vi "Aircraft Yaw Stability.vi"() -> ()   [LabVIEW 2022 SP3]
doc: "This example demonstrates how to continuously acquire buffered voltage measurements using a DAQmx device.\n\nFor instructions on how to connect your signals to the DAQ device, refer to your device documentation."
uses:
  <vilib>/Utility/error.llb/DialogType.ctl
  <vilib>/DAQmx/read.llb/DAQmx Read (Analog 1D Wfm NChan NSamp).vi
  <vilib>/DAQmx/create/channels.llb/DAQmx Create Channel (AI-Voltage-Basic).vi
  <vilib>/DAQmx/configure/timing.llb/DAQmx Timing (Sample Clock).vi
  <vilib>/DAQmx/configure/task.llb/DAQmx Configure Logging (TDMS).vi
  <vilib>/DAQmx/configure/trigger.llb/DAQmx Start Trigger (Digital Edge).vi
  <vilib>/DAQmx/configure/trigger.llb/DAQmx Start Trigger (Time).vi
  <vilib>/DAQmx/configure/trigger.llb/DAQmx Start Trigger (Analog Edge).vi
  <vilib>/DAQmx/miscellaneous.llb/DAQmx Fill In Error Info.vi
  <resource>/objmgr/daqmx.rc
panel:
  in  "File Name":string="Group1"
  in  "Folder":path=path "S:/Research/EnFlo_Data_Current/2024/A_Tunnel/UG Labs/Results/Res_12-2024"
  in  "Trigger Type":T1(tab)
  in  "Digital Start Trigger Edge":i32(ring)=10280 caption="Edge" items=["Rising"=10280, "Falling"=10171]
  in  "Digital Start Trigger Source":tag="/Dev1/PFI0" caption="Source"
  in  "Digital Pause Trigger Pause When":i32(ring)=10192 caption="Pause When" items=["High"=10192, "Low"=10214]
  in  "Digital Pause Trigger Source":tag="/Dev1/PFI0" caption="Source"
  in  "Analog Start Trigger Level":dbl caption="Level" format="%0.2f"
  in  "Analog Start Trigger Hysteresis":dbl caption="Hysteresis" format="%.2f"
  in  "Analog Start Trigger Slope":i32(ring)=10280 caption="Slope" items=["Rising"=10280, "Falling"=10171]
  in  "Analog Start Trigger Source":string="APFI0" caption="Source"
  in  "Analog Pause Trigger Source":string="APFI0" caption="Source"
  in  "Analog Pause Trigger Pause When":i32(ring)=10093 caption="Pause When" items=["Above Level"=10093, "Below Level"=10107]
  in  "Analog Pause Trigger Level":dbl caption="Level" format="%.2f"
  in  "When":timestamp
  in  "Select Time\nManually":bool
  in  "Stop":bool
  out "Waveform Chart":waveform(dbl)[](graph)
  in  "TDMS File Path":path
  in  "Number of Samples":i32=100
  in  "Sample Rate":dbl=1000.0
  in  "Sample Clock Source":tag="OnboardClock"
  in  "Terminal Configuration":i32(ring)=-1 items=["default"=-1, "RSE"=10083, "NRSE"=10078, "Differential"=10106, "Pseudodifferential"=12529]
  in  "Max Voltage":dbl=10.0
  in  "Min Voltage":dbl=-10.0
  in  "Physical Channel":tag="Dev1/ai0"
  out "Actual Sample Rate":dbl=1000.0 format="%0.2f"
  in  "Logging Mode":i32(ring)=10231 items=["Off"=10231, "Log and Read"=15842]
  # "Channel Settings"
  # "Timing Settings"
  # "Trigger Settings"
  # "Logging Settings"
  # "To enable triggers, select a tab above, and configure the settings.\n\nNot all hardware supports all trigger types. Refer to your device documentation for more information."
  # "This trigger type is not supported in continuous sample timing. \n\nRefer to your device documentation for more information on which triggers are supported."
  # "This trigger type is not supported in continuous sample timing. \n\nRefer to your device documentation for more information on which triggers are supported."
  # "If time is not manually set, task will begin after 10 seconds"
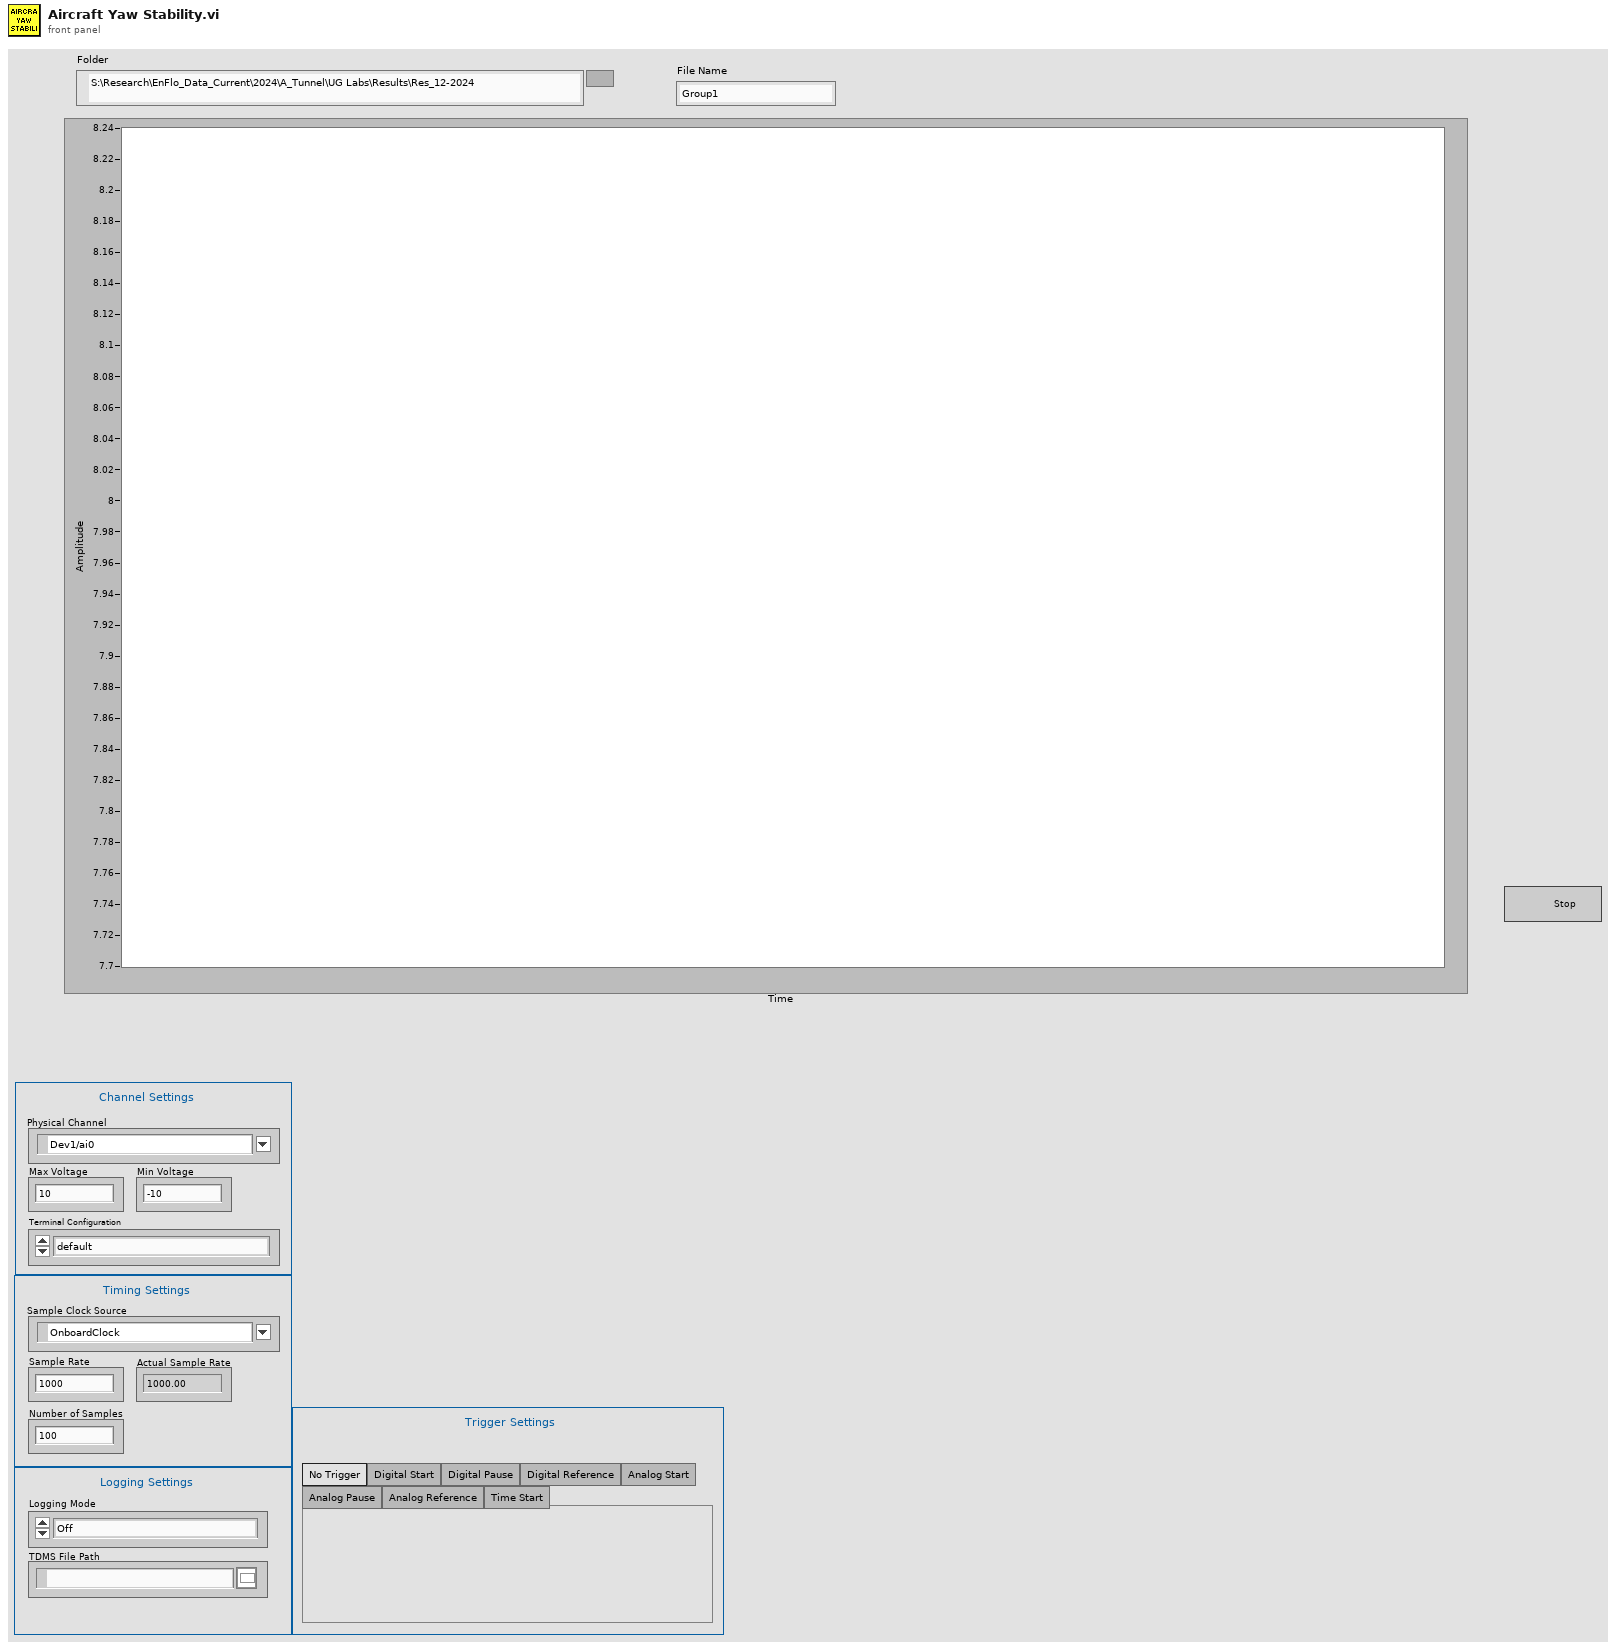
[diagram p1: front panel]
types:
  T1 = enum32{"No Trigger", "Digital Start", "Digital Pause", "Digital Reference", "Analog Start", "Analog Pause", "Analog Reference", "Time Start"}
  T2 = typedef "DialogType.ctl" = u16
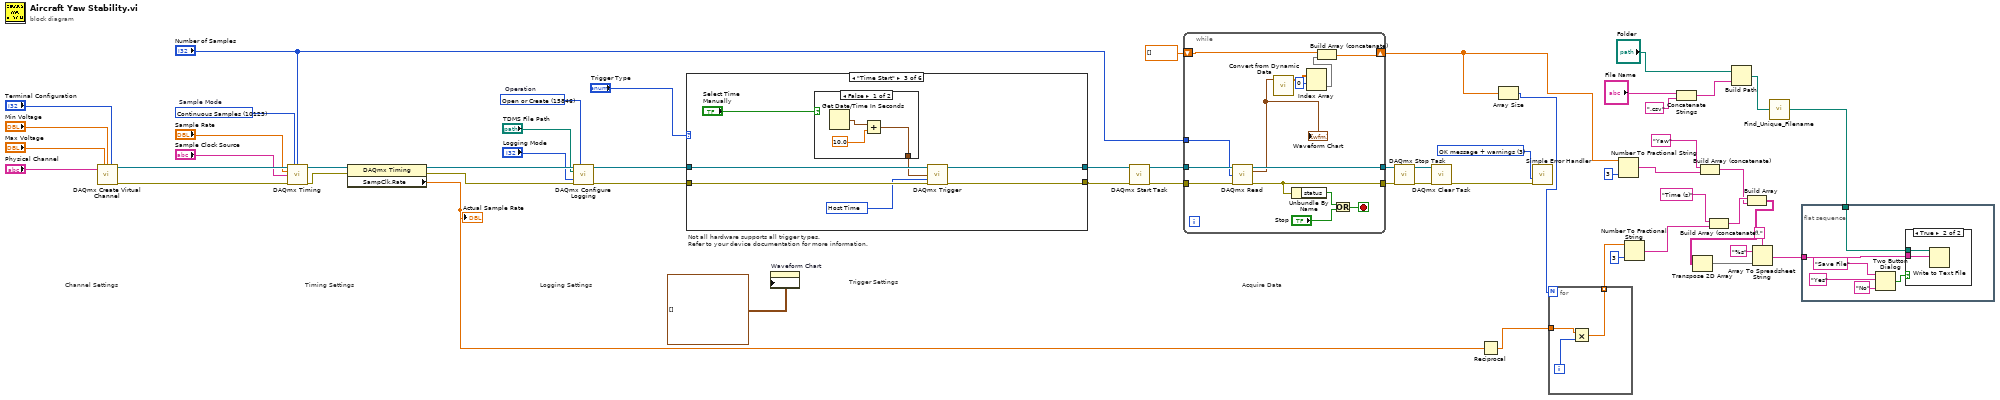
[diagram p0: block diagram]
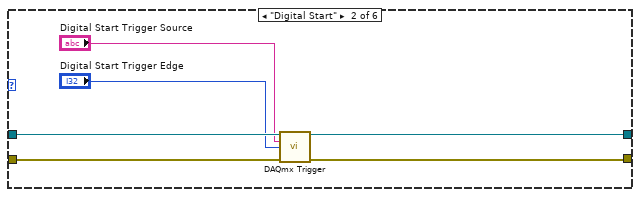
[diagram p4: hidden frame]
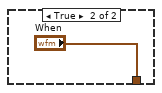
[diagram p5: hidden frame]
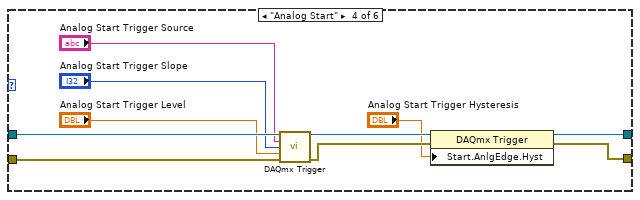
[diagram p6: hidden frame]
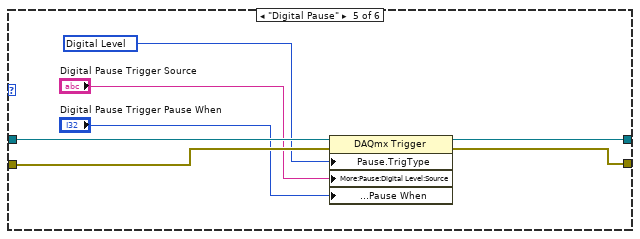
[diagram p7: hidden frame]
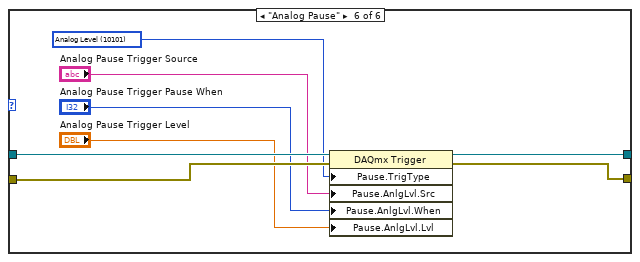
[diagram p8: hidden frame]
diagram:
  w32 = T2 3 items=["no dialog", "OK message", "continue or stop message", "OK message + warnings", "continue/stop + warnings"] ("type of dialog (OK msg:1)")
  w49 = 15846 items=["Open"=10437, "Open or Create"=15846, "Create or Replace"=15847, "Create"=15848]  # Operation
  w54 = 10123 items=["Finite Samples"=10178, "Continuous Samples"=10123, "Hardware Timed Single Point"=12522]  # Sample Mode
  # "Trigger Settings"
  # "Not all hardware supports all trigger types.\nRefer to your device documentation for more information."
  # "Acquire Data"
  # "Timing Settings"
  # "Channel Settings"
  # "Logging Settings"
  n1 = call-poly <vilib>:"DAQmx Create Virtual Channel.vi"("maximum value"="Max Voltage", "minimum value"="Min Voltage", "input terminal configuration"="Terminal Configuration", "physical channels"="Physical Channel") -> ("task out"=w52:refnum<k21>, "error out"=w53:errorcluster)  [unwired: 10 in]
  n2 = call-poly <vilib>:"DAQmx Timing.vi"("task/channels in"=w52, "sample mode"=w54, "samples per channel"="Number of Samples", "rate"="Sample Rate", "source"="Sample Clock Source", "error in"=w53) -> ("task out"=w56:refnum<k21>, "error out"=w55:errorcluster)  [unwired: 8 in]
  n3 = property class="DAQmx Timing"(reference=w56, error in=w55) -> (reference out=w51:refnum<k21>, error out=w50:errorcluster, "SampClk.Rate"=w25:dbl)
  "Actual Sample Rate" <- w25
  n4 = call-poly <vilib>:"DAQmx Configure Logging.vi"("task/channels in"=w51, "operation"=w49, "file path"="TDMS File Path", "logging mode"="Logging Mode", "error in"=w50) -> ("task out"=w30:refnum<k21>, "error out"=w29:errorcluster)  [unwired: 9 in]
  n5 = case shown="\"Time Start\"" "Trigger Type" {
    tunnel: w30 -> [w58 w64 w71 w85 w92 w100]
    tunnel: w29 -> [w57 w63 w70 w84 w89 w97]
    tunnel: [w58 w62 w69 w82 w91 w99] -> w27
    tunnel: [w57 w61 w68 w81 w90 w98] -> w28
    frame "No Trigger", Default {
    }
    frame "Digital Start" {
      n6 = call-poly <vilib>:"DAQmx Trigger.vi"("task/channels in"=w64, "source"="Digital Start Trigger Source", "edge"="Digital Start Trigger Edge", "error in"=w63) -> ("task out"=w62:refnum<k21>, "error out"=w61:errorcluster)  [unwired: 10 in]
    }
    frame "Time Start" {
      w67 = 16126 items=["Host Time"=16126, "I/O Device Time"=16127] ("timescale")
      n7 = case shown="False" "Select Time\nManually" {
        tunnel: [w72 "When"] -> w65
        frame False {
          n8 = Get Date/Time In Seconds() -> (seconds since 1Jan1904=w74:timestamp)
          n9 = Add(x=w74, y=10.0) -> (x+y=w72:timestamp)
        }
        frame True {
        }
      }
      n10 = call-poly <vilib>:"DAQmx Trigger.vi"("task/channels in"=w71, "when"=w65, "timescale"=w67, "error in"=w70) -> ("task out"=w69:refnum<k21>, "error out"=w68:errorcluster)  [unwired: 10 in]
    }
    frame "Analog Start" {
      n11 = call-poly <vilib>:"DAQmx Trigger.vi"("task/channels in"=w85, "source"="Analog Start Trigger Source", "slope"="Analog Start Trigger Slope", "level"="Analog Start Trigger Level", "error in"=w84) -> ("task out"=w80:refnum<k21>, "error out"=w79:errorcluster)  [unwired: 9 in]
      n12 = property class="DAQmx Trigger"(reference=w80, error in=w79, "Start.AnlgEdge.Hyst"="Analog Start Trigger Hysteresis") -> (reference out=w82:refnum<k21>, error out=w81:errorcluster)
    }
    frame "Digital Pause" {
      w88 = 10152 items=["Analog Level"=10101, "Analog Window"=10103, "Digital Level"=10152, "Digital Pattern"=10398, "None"=10230] ("Pause.TrigType")
      n13 = property class="DAQmx Trigger"(reference=w92, error in=w89, "Pause.TrigType"=w88, "More:Pause:Digital Level:Source"="Digital Pause Trigger Source", "More:Pause:Digital Level:Pause When"="Digital Pause Trigger Pause When") -> (reference out=w91:refnum<k21>, error out=w90:errorcluster)
    }
    frame "Analog Pause" {
      w96 = 10101 items=["Analog Level"=10101, "Analog Window"=10103, "Digital Level"=10152, "Digital Pattern"=10398, "None"=10230] ("Pause.TrigType")
      n14 = property class="DAQmx Trigger"(reference=w100, error in=w97, "Pause.TrigType"=w96, "Pause.AnlgLvl.Src"="Analog Pause Trigger Source", "Pause.AnlgLvl.When"="Analog Pause Trigger Pause When", "Pause.AnlgLvl.Lvl"="Analog Pause Trigger Level") -> (reference out=w99:refnum<k21>, error out=w98:errorcluster)
    }
  }
  n15 = property on="Waveform Chart" class="WFChart (strict)"("History Data"=waveform(dbl)[][] []) -> ()  [unwired: 2 in, 2 out]
  n16 = call <vilib>:"DAQmx Start Task.vi"("task/channels in"=w27, "error in"=w28) -> ("task out"=w48:refnum<k21>, "error out"=w47:errorcluster)  [unwired: 12 in]
  n17 = while {
    tunnel: w48 -> [w114]
    tunnel: w47 -> [w113]
    tunnel: [w112] -> w36
    tunnel: [w110] -> w35
    tunnel: "Number of Samples" -> [w107]
    shift-right: [w105] -> w18
    shift-left: dbl[] [] -> [w106]
    stop <- w108 stop-if-true
    n18 = call-poly <vilib>:"DAQmx Read.vi"("task/channels in"=w114, "number of samples per channel"=w107, "error in"=w113) -> ("task out"=w112:refnum<k21>, "data"=w104:waveform(dbl)[], "error out"=w110:errorcluster)  [unwired: 10 in]
    "Waveform Chart" <- w104
    n19 = call "Convert from Dynamic Data"("Dynamic Data Type"=w104) -> ("Array"=w103:dbl[][])  [unwired: 3 in]
    n20 = Unbundle By Name(w110) -> ("status"=w109:bool)
    n21 = Index Array(array=w103, index (row)=0) -> (element=w101:dbl[])  [unwired: 1 in]
    n22 = Build Array (concatenate)(w106, w101) -> (w105:dbl[])
    n23 = Or(x=w109, y="Stop") -> (x .or. y?=w108:bool)
  }
  n24 = call <vilib>:"DAQmx Stop Task.vi"("task/channels in"=w36, "error in"=w35) -> ("task out"=w33:refnum<k21>, "error out"=w34:errorcluster)  [unwired: 12 in]
  n25 = call <vilib>:"DAQmx Clear Task.vi"("task in"=w33, "error in"=w34) -> ("error out"=w46:errorcluster)  [unwired: 13 in]
  n26 = Reciprocal(x=w25) -> (1/x=w23:dbl)
  n27 = Array Size(array=w18) -> (size(s)=w24:i32)
  n28 = call <vilib>:"Simple Error Handler.vi"("type of dialog (OK msg:1)"=w32, "error in (no error)"=w46) -> ()  [unwired: 3 in, 5 out]
  n29 = for {
    N: w24 -> [_]
    tunnel: w23 -> [w116]
    tunnel: [w115] -> w13 mode=indexing
    i -> [w117]
    n30 = Multiply(x=w116, y=w117) -> (x*y=w115:dbl)
  }
  n31 = Number To Fractional String(number=w18, precision (6)=i16 3) -> (F-format string=w16:string[])  [unwired: 2 in]
  n32 = Number To Fractional String(number=w13, precision (6)=i16 3) -> (F-format string=w11:string[])  [unwired: 2 in]
  n33 = Concatenate Strings("File Name", ".csv" ("string")) -> (w4:string)
  n34 = Build Array (concatenate)("Yaw", w16) -> (w9:string[])
  n35 = Build Array (concatenate)("Time (s)", w11) -> (w10:string[])
  n36 = Build Path(base path="Folder", name or relative path=w4) -> (appended path=w3:path)
  n37 = Build Array(w10, w9) -> (w8:string[][])
  n38 = Transpose 2D Array(2D array=w8) -> (transposed array=w19:string[][])
  n39 = Array To Spreadsheet String(delimiter (Tab)=",", array=w19, 3:"%s" ("format string")) -> (spreadsheet string=w21:string)
  n40 = call "Find_Unique_Filename.vi"("Path In"=w3) -> ("Unique Path Out"=w2:path)  [unwired: 2 in]
  n41 = flat-sequence {
    tunnel: w21 -> [w123]
    tunnel: w2 -> [w122]
    frame #0 {
      n42 = Two Button Dialog(message="Save File", 1:"No" ("F button name (\"Cancel\")"), 2:"Yes" ("T button name (\"OK\")")) -> (T button?=w119:bool)
      n43 = case shown="True" w119 {
        tunnel: w123 -> [_ w125]
        tunnel: w122 -> [_ w124]
        frame False {
        }
        frame True {
          n44 = Write to Text File(file (use dialog)=w124, text=w125) -> ()  [unwired: 2 in, 3 out]
        }
      }
    }
  }
